vi "Two-Point Linear Interpolation.vi"(3 "x":dbl format="%.2f", 4 "X":dbl[](array[numeric]) format="%.2f", 5 "Y":dbl[](array[numeric]) format="%.2f") -> (2 "interpolation value":dbl format="%.2f")   [LabVIEW 2011]
doc: "Interpolates the function f at x, given a set of n points {x(i),y(i)} where f(x(i))=y(i), f is any function and x is in the range of x(i).\nThe VI caculates output interpolation value based on a two-point interpolation about the closest neighboring \"Y\" values..\n\nThe \"X\" array must be in ascending (increasing) value order."
panel:
  # "2 Point Linear Interpolation"
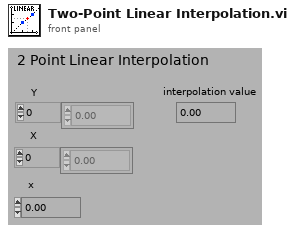
[diagram p1: front panel]
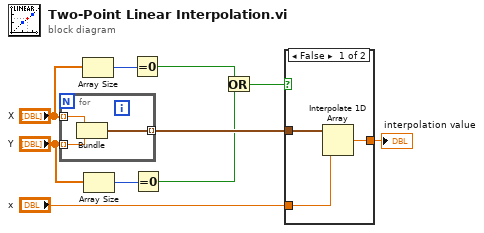
[diagram p0: block diagram]
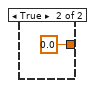
[diagram p2: hidden frame]
diagram:
  n1 = for {
    tunnel: "X" -> [w13] mode=indexing
    tunnel: "Y" -> [w12] mode=indexing
    tunnel: [w11] -> w10 mode=indexing
    n2 = Bundle(w13, w12) -> (w11:cluster{dbl, dbl})  [unwired: 1 out]
  }
  n3 = Array Size(array="X") -> (size(s)=w7:i32)
  n4 = Array Size(array="Y") -> (size(s)=w5:i32)
  n5 = Equal To 0?(x=w7) -> (x = 0?=w6:bool)
  n6 = Equal To 0?(x=w5) -> (x = 0?=w2:bool)
  n7 = Or(x=w6, y=w2) -> (x .or. y?=w1:bool)
  n8 = case shown="False" w1 {
    tunnel: w10 -> [w16 _]
    tunnel: "x" -> [w15 _]
    tunnel: [w14 0.0] -> w8
    frame False {
      n9 = Interpolate 1D Array(1:w15, 2:w16) -> (0:w14:dbl)
    }
    frame True {
    }
  }
  "interpolation value" <- w8
